vi "Clean up.vi"(8 "error in (no error)":errorcluster, 11 "Analyze BaseClass in":refnum<class "Analyze BaseClass.lvclass">) -> (0 "error out":errorcluster, 3 "Analyze BaseClass out":refnum<class "Analyze BaseClass.lvclass">)   [LabVIEW 2020, in "Analyze.lvlib" / "Analyze BaseClass.lvlib" / "Analyze BaseClass.lvclass"]
uses:
  Analyze BaseClass.lvclass
  Analyze BaseClass.lvclass/Analyze BaseClass.ctl
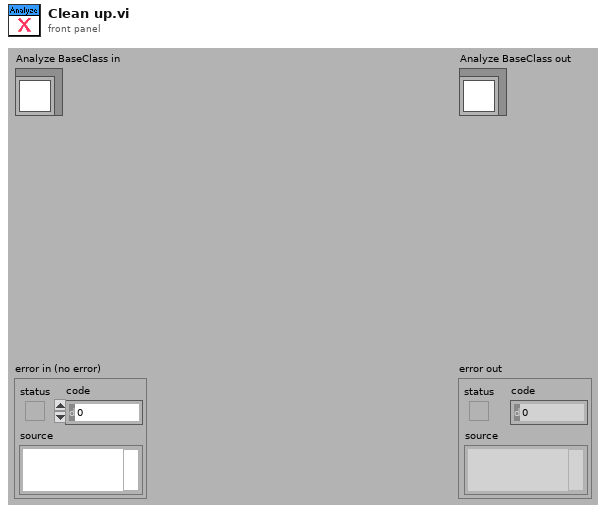
[diagram p1: front panel]
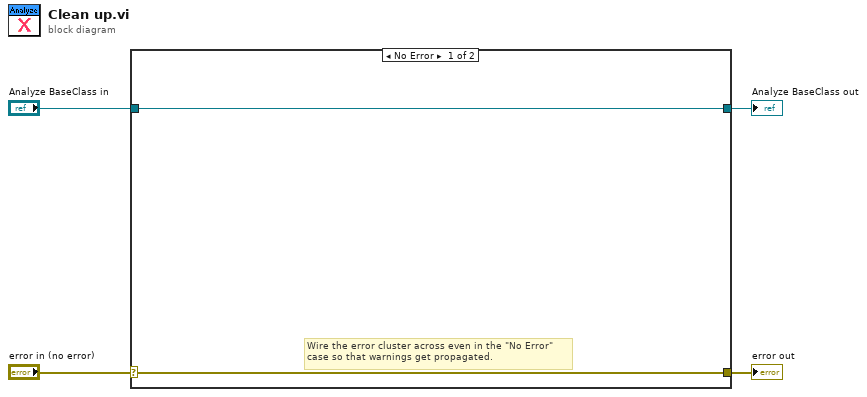
[diagram p0: block diagram]
diagram:
  n1 = case shown="No Error" "error in (no error)" {
    selector: "error in (no error)" -> [w5 w8]
    tunnel: [w5 w8] -> w3
    tunnel: [w6 w7] -> w1
    tunnel: "Analyze BaseClass in" -> [w6 w7]
    frame No Error {
      # "Wire the error cluster across even in the \"No Error\"\ncase so that warnings get propagated."
    }
    frame Error {
    }
  }
  "error out" <- w3
  "Analyze BaseClass out" <- w1
